vi "Driverstation.vi"   [LabVIEW 2012]
uses:
  Robot Global Data.vi
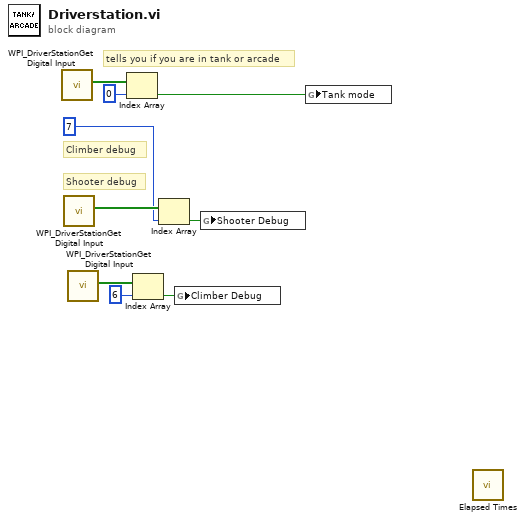
[diagram p0: block diagram]
diagram:
  # "Climber debug"
  # "Shooter debug"
  # "tells you if you are in tank or arcade"
  n1 = call <vilib>:"WPI_DriverStationGet Digital Input.vi"() -> ("Driver Station Digital Input (1-8)"=w9:bool[])  [unwired: 11 in]
  n2 = call <vilib>:"WPI_DriverStationGet Digital Input.vi"() -> ("Driver Station Digital Input (1-8)"=w6:bool[])  [unwired: 11 in]
  n3 = call <vilib>:"WPI_DriverStationGet Digital Input.vi"() -> ("Driver Station Digital Input (1-8)"=w2:bool[])  [unwired: 11 in]
  n4 = Index Array(array=w9, index=0) -> (element=w7:bool)
  n5 = Index Array(array=w2, index=6) -> (element=w1:bool)
  n6 = Index Array(array=w6, index=7) -> (element=w4:bool)
  n7 = global write "Robot Global Data.vi" "Climber Debug"(w1) -> ()
  n8 = global write "Robot Global Data.vi" "Shooter Debug"(w4) -> ()
  n9 = global write "Robot Global Data.vi" "Tank mode"(w7) -> ()
  n10 = call "Elapsed Times.vi"() -> ()  [unwired: 3 in, 1 out]
